vi "Do.vi"(8 "error in (no error)":errorcluster, 10 "Actor in":refnum<class "Actor.lvclass">, 11 "Check Validity of Selection.lvclass":refnum<class "Check Validity of Selection.lvclass">) -> (0 "error out":errorcluster, 2 "Actor out":refnum<class "Actor.lvclass">)   [LabVIEW 2016, in "Controller UI.lvlib" / "Check Validity of Selection.lvclass"]
uses:
  <userlib>/Common Components/Controller UI/Messages/Check Run Button/Check Validity of Selection.lvclass
  <vilib>/ActorFramework/Actor/Actor.lvclass
  <userlib>/Common Components/Controller UI/Controller UI.lvclass
  C:/Program Files (x86)/National Instruments/LabVIEW 2016/vi.lib/ActorFramework/Actor/Actor.lvclass
  <userlib>/Common Components/Controller UI/Messages/Check Run Button/Check Validity of Selection.lvclass/Check Validity of Selection.ctl
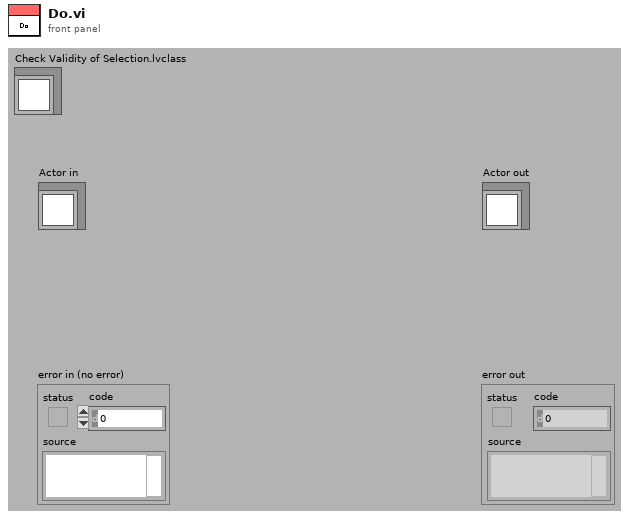
[diagram p1: front panel]
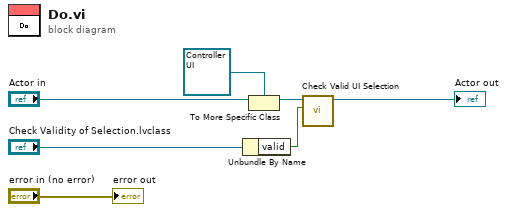
[diagram p0: block diagram]
diagram:
  n1 = Unbundle By Name("Check Validity of Selection.lvclass") -> ("valid"=w1:bool)
  n2 = To More Specific Class(target class=refnum<class "Controller UI.lvclass"> refnum ("UI.lvclass"), reference="Actor in") -> (specific class reference=w4:refnum<class "Controller UI.lvclass">)  [unwired: 1 in, 1 out]
  n3 = call-dynamic "Check Valid UI Selection.vi"("valid"=w1, "Operator UI in"=w4) -> ("Operator UI out"=→"Actor out":refnum<class "Controller UI.lvclass">)  [unwired: 8 in, 1 out]
  "error out" <- "error in (no error)"
